vi "calc.vi"(3 "Acquire":refnum<vi>, 4 "filter":bool caption="Фильтр включен", 5 "ArrayIn":waveform(i16)[](array[waveform])) -> (0 "AllMeasures":cluster{"x0":dbl, "dx":dbl, "y":sgl[][]}[](array[cluster]), 2 "Values":string[][](array[string]))   [LabVIEW 2010]
uses:
  70user.lib/TheSigTab.vi
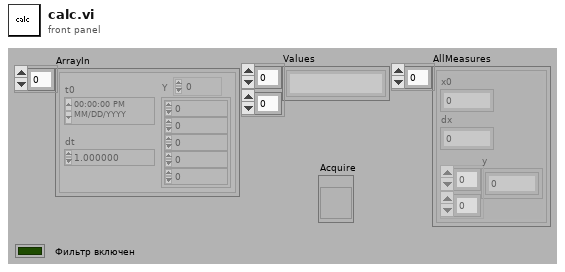
[diagram p1: front panel]
types:
  T1 = enum16{"Напряжение/Ток", "ЧР", "Температура", "Давление"}
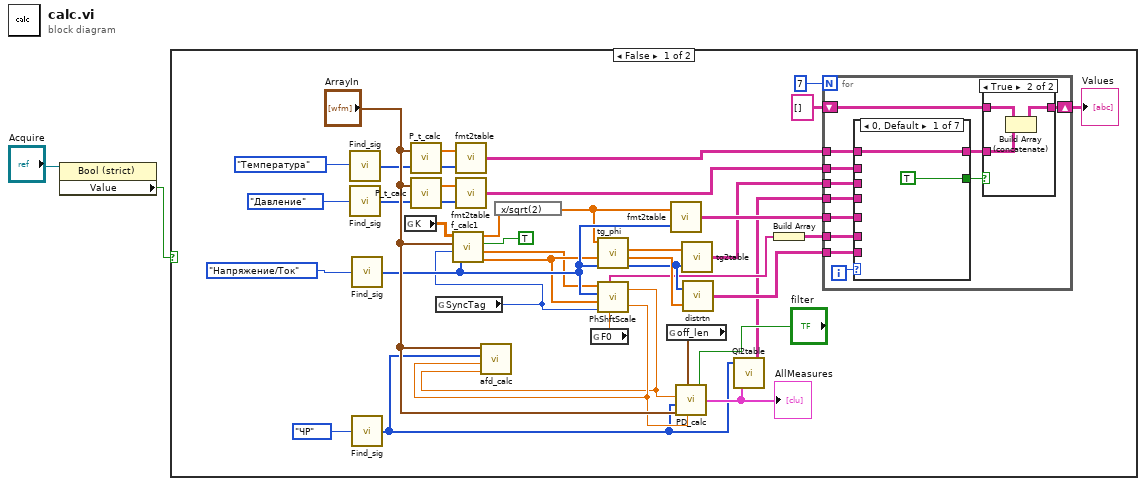
[diagram p0: block diagram]
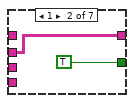
[diagram p3: hidden frame]
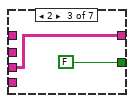
[diagram p4: hidden frame]
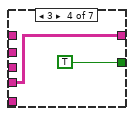
[diagram p5: hidden frame]
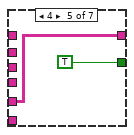
[diagram p6: hidden frame]
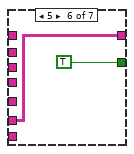
[diagram p7: hidden frame]
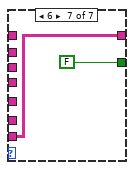
[diagram p8: hidden frame]
diagram:
  n1 = property class="Bool (strict)"(reference="Acquire") -> ("Value"=w1:bool)  [unwired: 1 in, 2 out]
  n2 = case shown="False" w1 {
    frame False {
      n3 = call "Find_sig.vi"("Тип"=T1."Температура") -> ("Indexies"=w24:i32[])
      n4 = call "Find_sig.vi"("Тип"=T1."Давление") -> ("Indexies"=w26:i32[])
      n5 = call "Find_sig.vi"("Тип"=T1."Напряжение/Ток") -> ("Indexies"=w33:i32[])
      n6 = call "Find_sig.vi"("Тип"=T1."ЧР") -> ("Indexies"=w19:i32[])
      n7 = global read "TheSigTab.vi" "K"() -> (w15:dbl[][])
      n8 = call "P_t_calc.vi"("Indexies"=w24, "Array"="ArrayIn") -> ("Indexies 2"=w27:i32[], "Array 2"=w23:sgl[])
      n9 = call "P_t_calc.vi"("Indexies"=w26, "Array"="ArrayIn") -> ("Indexies 2"=w28:i32[], "Array 2"=w25:sgl[])
      n10 = global read "TheSigTab.vi" "SyncTag"() -> (w16:i32)
      n11 = call "f_calc1.vi"("Reset"=TRUE ("reset"), "Indx"=w33, "SyncTag"=w16, "Array"="ArrayIn", "K"=w15) -> ("Phases"=w31:dbl[], "Freqs"=w29:dbl[], "Amps"=w34:dbl[])
      n12 = call "fmt2table.vi"("Tags"=w27, "Array 2"=w23) -> ("Table"=w7:string[][])
      n13 = call "fmt2table.vi"("Tags"=w28, "Array 2"=w25) -> ("Table"=w8:string[][])
      n14 = expression code="x/sqrt(2)"(w34) -> (w22:dbl[])
      n15 = global read "TheSigTab.vi" "F0"() -> (w30:dbl)
      n16 = call "tg_phi.vi"("Tags"=w33, "detected phases (deg)"=w31, "RMS"=w22) -> ("Tags 2"=w18:i32[], "G"=w21:cdb[], "tg"=w32:dbl[])  [unwired: 4 in]
      n17 = call "PhShftScale.vi"("F0"=w30, "SyncTag"=w16, "detected phase (deg)"=w31, "Tags"=w33, "detected frequency"=w29) -> ("delay"=w37:dbl, "T"=w36:dbl, "Table"=w14:string[])
      n18 = call "afd_calc.vi"("Array"="ArrayIn", "Indexies"=w19, "TStart"=w37, "T"=w36) -> ()  [unwired: 1 in, 1 out]
      n19 = global read "TheSigTab.vi" "off_len"() -> (w20:cluster{"offset":dbl, "length":dbl}[])
      n20 = call "fmt2table.vi"("Tags"=w33, "Array 2"=w22) -> ("Table"=w11:string[][])
      n21 = call "PD_calc.vi"("off_len"=w20, "T(sec)"=w36, "list"=w19, "tStart"=w37, "ArrayIn"="ArrayIn", "filter"="filter") -> ("AllMeasures"=w35:cluster{"x0":dbl, "dx":dbl, "y":sgl[][]}[])  [unwired: 2 out]
      "AllMeasures" <- w35
      n22 = call "tg2table.vi"("Tags"=w18, "Array 2"=w32) -> ("Table"=w9:string[][])
      n23 = call "distrtn.vi"("G"=w21, "indxs"=w18) -> ("Array"=w13:string[][])
      n24 = call "QI2table.vi"("Array In"=w35, "Indexies"=w19) -> ("Array"=w10:string[][])  [unwired: 1 in]
      n25 = Build Array(w14) -> (w12:string[][])
      n26 = for {
        N: 7 -> [_]
        tunnel: w13 -> [w54]
        tunnel: w12 -> [w53]
        tunnel: w11 -> [w52]
        tunnel: w10 -> [w51]
        tunnel: w9 -> [w50]
        tunnel: w8 -> [w49]
        tunnel: w7 -> [w48]
        shift-right: [w46] -> w4
        shift-left: string[][] [] -> [w45]
        i -> [w44]
        n27 = case shown="0, Default" w44 {
          tunnel: w54 -> [_ _ _ _ _ _ w72]
          tunnel: w53 -> [_ _ _ _ _ w70 _]
          tunnel: w52 -> [_ _ _ _ w68 _ _]
          tunnel: w51 -> [_ _ _ w66 _ _ _]
          tunnel: w50 -> [_ _ w64 _ _ _ _]
          tunnel: w49 -> [_ w62 _ _ _ _ _]
          tunnel: w48 -> [w60 _ _ _ _ _ _]
          tunnel: [w60 w62 w64 w66 w68 w70 w72] -> w47
          tunnel: [TRUE ("filter") TRUE ("filter") FALSE ("filter") TRUE ("filter") TRUE ("filter") TRUE ("filter") FALSE ("filter")] -> w43
          frame 0, Default {
          }
          frame 1 {
          }
          frame 2 {
          }
          frame 3 {
          }
          frame 4 {
          }
          frame 5 {
          }
          frame 6 {
          }
        }
        n28 = case shown="True" w43 {
          tunnel: w47 -> [_ w58]
          tunnel: [w55 w57] -> w46
          tunnel: w45 -> [w55 w56]
          frame False {
          }
          frame True {
            n29 = Build Array (concatenate)(w56, w58) -> (w57:string[][])
          }
        }
      }
      "Values" <- w4
    }
    frame True {
    }
  }
